vi "HEWH Find 60 Seconds Before.vi"(8 "error in (no error)":errorcluster, 9 "Software Elapsed Time (sec)":dbl[](array[numeric]) format="%#.6g", 10 "Elapsed Time (sec)":dbl[](array[numeric]) format="%#.6g", 11 "Start Index":i32) -> (0 "error out":errorcluster, 3 "Index (60 Seconds Before)":i32)   [LabVIEW 2023]
panel:
  out "Search Element":dbl
  out "Start Time":dbl
  out "Target Time":dbl
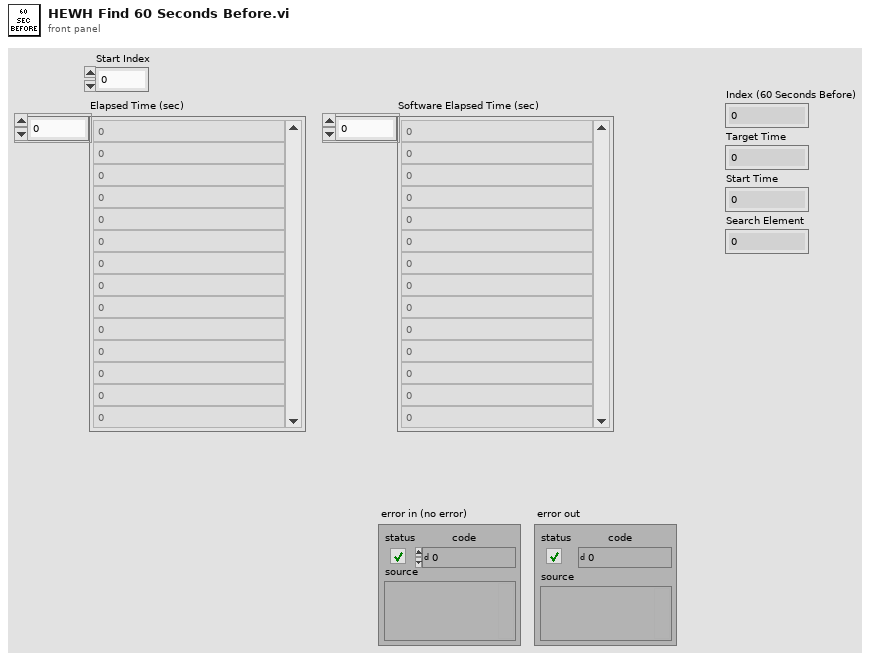
[diagram p1: front panel]
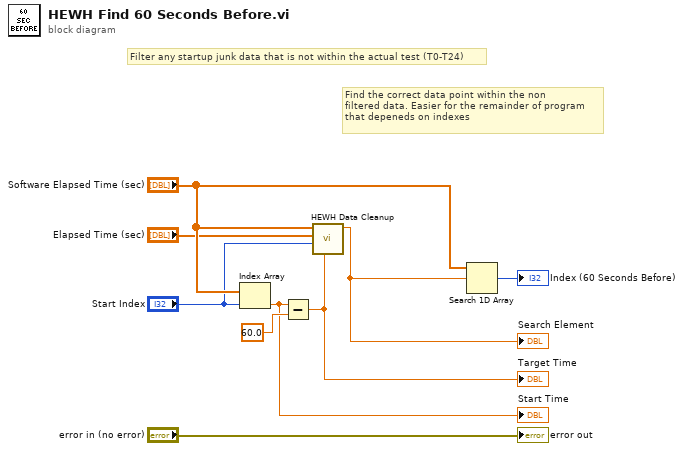
[diagram p0: block diagram]
diagram:
  # "Find the correct data point within the non\nfiltered data. Easier for the remainder of program\nthat depeneds on indexes"
  # "Filter any startup junk data that is not within the actual test (T0-T24)"
  n1 = Index Array(array="Software Elapsed Time (sec)", index="Start Index") -> (element=w3:dbl)
  "Start Time" <- w3
  n2 = Subtract(x=w3, y=60.0) -> (x-y=w2:dbl)
  "Target Time" <- w2
  n3 = call "HEWH Data Cleanup.vi"("60 Second Before Start"=w2, "Start Index"="Start Index", "Elapsed Time (sec)"="Elapsed Time (sec)", "Software Elapsed Time (sec)"="Software Elapsed Time (sec)") -> ("Search Element"=w1:dbl)  [unwired: 6 in, 1 out]
  "Search Element" <- w1
  n4 = Search 1D Array(1D array="Software Elapsed Time (sec)", element=w1) -> (index of element=→"Index (60 Seconds Before)":i32)  [unwired: 1 in]
  "error out" <- "error in (no error)"
